vi "TP 2.1 (con variable t).vi"() -> ()   [LabVIEW 2013]
panel:
  in  "stop":bool
  out "Waveform Graph":dbl[](graph)
  in  "Amplitud":dbl
  in  "Frecuencia":dbl
  in  "Cantida de Muestras":dbl
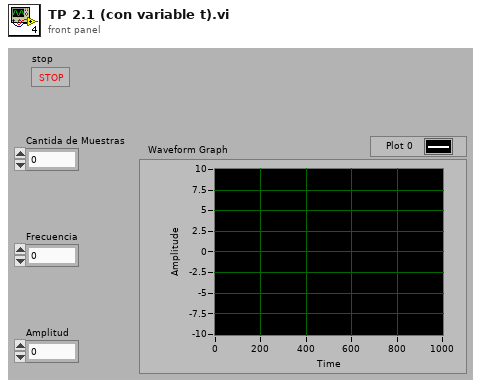
[diagram p1: front panel]
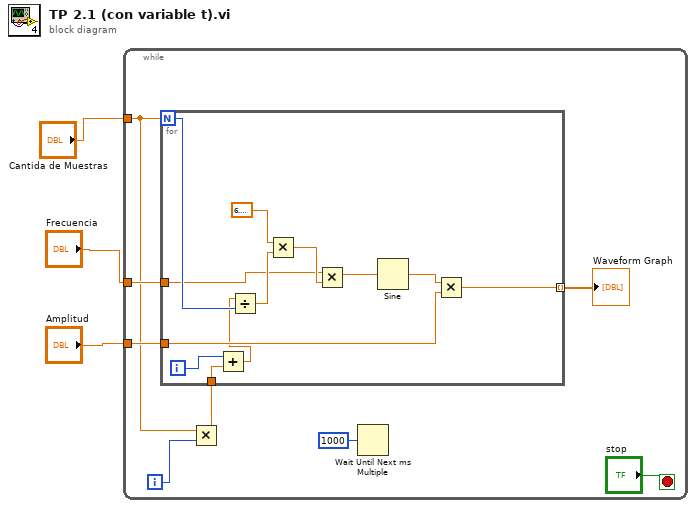
[diagram p0: block diagram]
diagram:
  n1 = while {
    tunnel: "Cantida de Muestras" -> [w5]
    tunnel: "Frecuencia" -> [w11]
    tunnel: "Amplitud" -> [w10]
    i -> [w6]
    stop <- "stop" stop-if-true
    n2 = Multiply(x=w5, y=w6) -> (x*y=w4:dbl)
    n3 = for {
      N: w5 -> [w23]
      tunnel: w11 -> [w20]
      tunnel: w10 -> [w16]
      tunnel: [w15] -> w9 mode=indexing
      tunnel: w4 -> [w14]
      i -> [w13]
      n4 = Add(x=w13, y=w14) -> (x+y=w12:dbl)
      n5 = Divide(x=w12, y=w23) -> (x/y=w22:dbl)
      n6 = Multiply(x=6.283185307179586, y=w22) -> (x*y=w21:dbl)
      n7 = Multiply(x=w20, y=w21) -> (x*y=w18:dbl)
      n8 = Sine(x=w18) -> (sin(x)=w17:dbl)
      n9 = Multiply(x=w17, y=w16) -> (x*y=w15:dbl)
    }
    "Waveform Graph" <- w9
    n10 = Wait Until Next ms Multiple(millisecond multiple=u32 1000) -> ()  [unwired: 1 out]
  }
